vi "backup init.vi"(4 "ref dest":u64, 8 "error in (no error)":errorcluster, 10 "ref src":u64) -> (0 "error out":errorcluster, 3 "backup_ref":u64)   [LabVIEW 2020, in "sqlite3.lvlib"]
uses:
  sqlite3.lvlib
  bin/sqlite3_64.dll
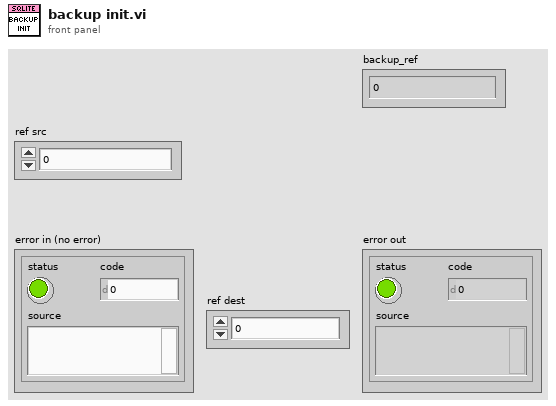
[diagram p1: front panel]
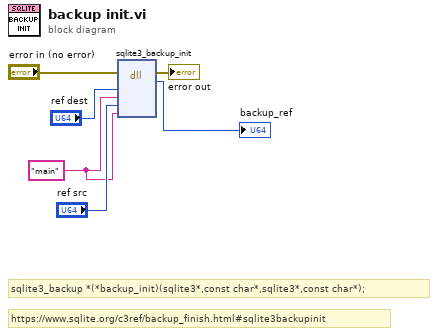
[diagram p0: block diagram]
diagram:
  w1 = "main" ("name dest")
  # "https://www.sqlite.org/c3ref/backup_finish.html#sqlite3backupinit"
  # "sqlite3_backup *(*backup_init)(sqlite3*,const char*,sqlite3*,const char*);"
  n1 = dll-call lib="D:/Project/Labview-Projects/database-configuration/externals/sqlite3/Source/bin/sqlite3_*.*" fn="sqlite3_backup_init"(error in="error in (no error)", "ref dest"="ref dest", "name dest"=w1, "ref src"="ref src", "name scr"=w1) -> (error out=→"error out":errorcluster, "return type"=→"backup_ref":u64)  [unwired: 6 in, 1 out]
